vi "New Segmented Log (No Limit).vi"(8 "error in (no error)":errorcluster, 9 "Max Instances (1)":i32=1, 11 "Log File Specification":refnum<class "Log File Specification.lvclass">) -> (0 "error out":errorcluster, 3 "Segmented Log out":refnum<class "Segmented Log.lvclass">)   [LabVIEW 2012, in "Waveform Data Logger Engine.lvlib" / "Segmented Log.lvclass"]
uses:
  Segmented Log.lvclass
  Shared/Classes/Log File Specifications/Log File Specification/Log File Specification.lvclass
  Segmented Log.lvclass/Segmented Log.ctl
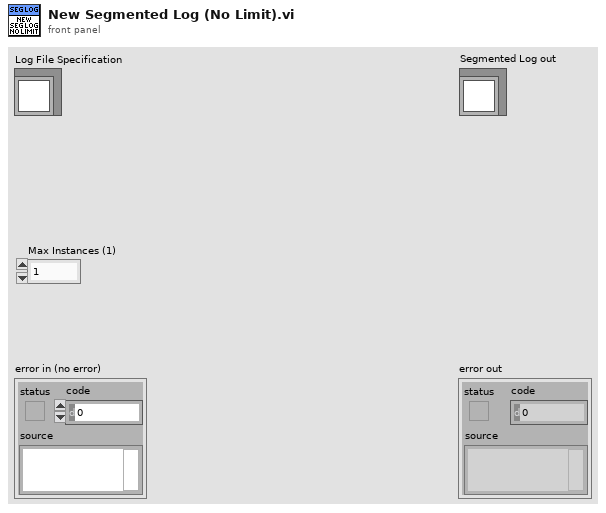
[diagram p1: front panel]
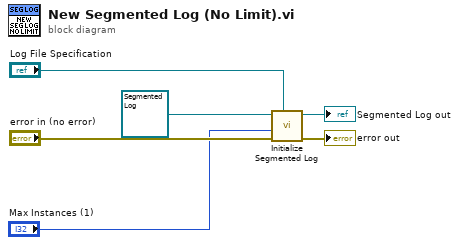
[diagram p0: block diagram]
diagram:
  n1 = call "Initialize Segmented Log.vi"("Log File Specification"="Log File Specification", "error in (no error)"="error in (no error)", "Max Instances (1)"="Max Instances (1)", "Segmented Log in"=refnum<class "Segmented Log.lvclass"> refnum ("Segmented Log out")) -> ("error out"=→"error out":errorcluster, "Segmented Log out"=→"Segmented Log out":refnum<class "Segmented Log.lvclass">)  [unwired: 6 in]
